vi "expansor_y_kaisser.vi"(6 "delta (rizado)":dbl, 9 "Banda Transicion (normalizada)":dbl, 10 "I factor interpolación":i32, 11 "Array":dbl[](array[numeric])) -> (3 "Filtered X":dbl[](array[numeric]))   [LabVIEW 2020]
uses:
  <vilib>/Analysis/3filter.llb/Filter Passband Type.ctl
  <vilib>/Analysis/4window.llb/windowTd.ctl
  <vilib>/Analysis/2dsp.llb/Upsample (DBL).vi
  <vilib>/Analysis/3filter.llb/FIR Filter (DBL).vi
  <vilib>/Analysis/NI_AALPro.lvlib
  <vilib>/Analysis/NI_AALBase.lvlib
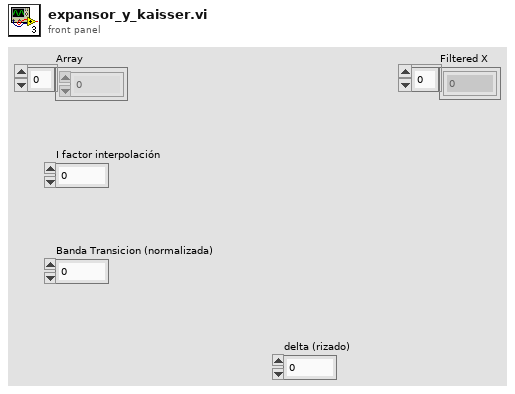
[diagram p1: front panel]
types:
  T1 = typedef "NI_AALPro.lvlib/windowTd.ctl" = u32
  T2 = typedef "NI_AALBase.lvlib/Filter Passband Type.ctl" = enum32{"Lowpass", "Highpass", "Bandpass", "Bandstop"}
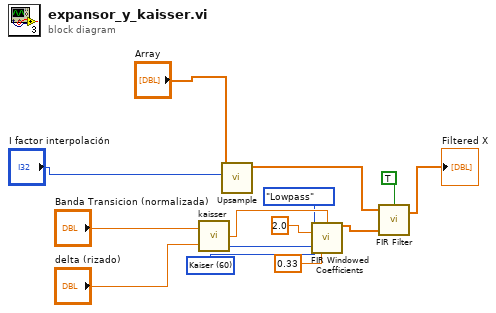
[diagram p0: block diagram]
diagram:
  w10 = T1 60 items=["Rectangle"=0, "Hanning"=1, "Hamming"=2, "Blackman-Harris"=3, "Exact Blackman"=4, "Blackman"=5, "Flat Top"=6, "4 Term B-Harris "=7, "7 Term B-Harris"=8, "Low Sidelobe"=9, "Blackman Nuttall"=11, "Triangle"=30, "Bartlett-Hanning"=31, "Bohman"=32, "Parzen"=33, "Welch"=34, "Kaiser"=60, "Dolph-Chebyshev"=61, "Gaussian"=62] ("window")
  n1 = call "kaisser.vi"("Banda Transicion (normalizada)"="Banda Transicion (normalizada)", "delta (rizado)"="delta (rizado)") -> ("Beta"=w9:dbl, "N+1"=w6:i32)  [unwired: 1 out]
  n2 = call-poly <vilib>:"Upsample.vi"("upsampling factor"="I factor interpolación", "X"="Array") -> ("Upsampled Array"=w12:dbl[])  [unwired: 8 in, 1 out]
  n3 = call <vilib>:"FIR Windowed Coefficients.vi"("filter type"=Filter_Passband_Type."Lowpass", "window parameter"=w9, "sampling freq: fs"=2.0, "taps"=w6, "window"=w10, "low cutoff freq: fl"=0.33) -> ("FIR Windowed Coefficients"=w11:dbl[])  [unwired: 8 in, 1 out]
  n4 = call-poly <vilib>:"FIR Filter.vi"("init/cont (init:F)"=TRUE, "FIR Coefficients"=w11, "X"=w12) -> ("Filtered X"=→"Filtered X":dbl[])  [unwired: 1 in, 1 out]
